vi "FTW-Scheduler-Destroy.vi"(0 "FTW Job Scheduler":refnum<class "FTW-Scheduler.lvclass">, 11 "error in":errorcluster) -> (6 "Remaining Jobs":string, 15 "error out":errorcluster)   [LabVIEW 2015, in "FTW-Scheduler.lvclass"]
uses:
  FTW-Scheduler.lvclass
  json/FTW-JSON-Type.ctl
  codegen/xnode/FTW-JSON-Fetch.xnode
  core/type/FTW-Type-JSON.ctl
panel:
  out "Statistics":string
  # "Inputs"
  # "Outputs"
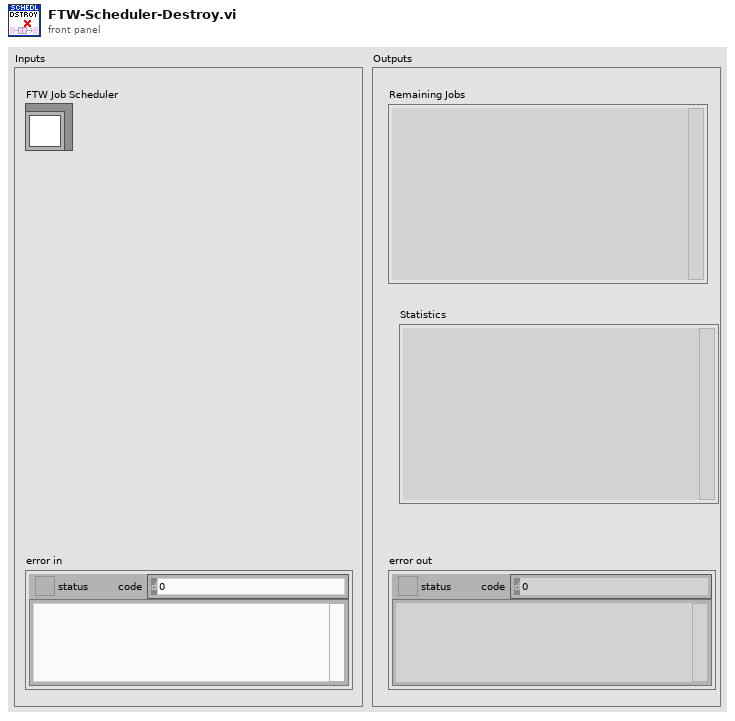
[diagram p1: front panel]
types:
  T1 = typedef "FTW-Type-JSON.ctl" = refnum<data-value>
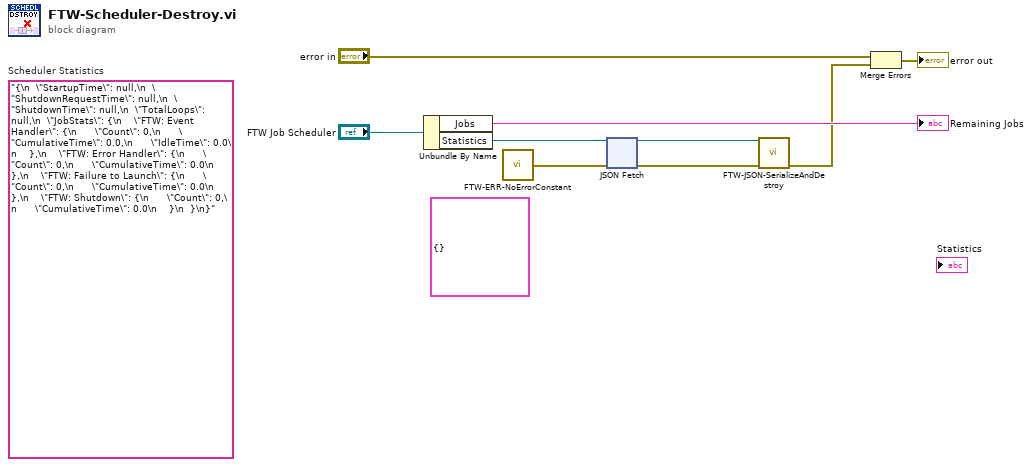
[diagram p0: block diagram]
diagram:
  (unwired) cluster{} {}
  (unwired) "{\n  \"StartupTime\": null,\n  \"ShutdownRequestTime\": null,\n  \"ShutdownTime\": null,\n  \"TotalLoops\": null,\n  \"JobStats\": {\n    \"FTW: Event Handler\": {\n      \"Count\": 0,\n      \"CumulativeTime\": 0.0,\n      \"IdleTime\": 0.0\n    },\n    \"FTW: Error Handler\": {\n      \"Count\": 0,\n      \"CumulativeTime\": 0.0\n    },\n    \"FTW: Failure to Launch\": {\n      \"Count\": 0,\n      \"CumulativeTime\": 0.0\n    },\n    \"FTW: Shutdown\": {\n      \"Count\": 0,\n      \"CumulativeTime\": 0.0\n    }\n  }\n}"  # Scheduler Statistics
  n1 = Unbundle By Name("FTW Job Scheduler") -> ("Jobs"=→"Remaining Jobs":string, "Statistics"=w4:T1)
  n2 = call "FTW-ERR-NoErrorConstant.vi"() -> ("no error"=w2:errorcluster)
  n3 = xnode "JSON Fetch"("JSON"=w4, "error in"=w2) -> ("JSON out"=w3:T1, "error out"=w1:errorcluster)  [unwired: 3 in, 2 out]
  n4 = call "FTW-JSON-SerializeAndDestroy.vi"("JSON"=w3, "error in"=w1) -> ("error out"=w5:errorcluster)  [unwired: 12 in, 1 out]
  n5 = Merge Errors("error in", w5) -> (→"error out":errorcluster)
